vi "2DRandomInterp.vi"() -> ()   [LabVIEW 2016]
uses:
  <vilib>/gmath/interp.llb/Interpolate 2D (2d X,Y).vi
  <vilib>/picture/3D Picture Control/Object/Create Object (drawable).vi
  <vilib>/picture/3D Picture Control/Helpers/Apply Texture (no reference).vi
  <vilib>/gmath/NI_Gmath.lvlib
  <vilib>/picture/3D Picture Control/NI_3D Picture Control.lvlib
  <vilib>/picture/3D Picture Control/Object/Add Object (no reference).vi
panel:
  out "3D Picture":refnum<vi>(3d-picture)
  in  "x":i32
  in  "y":i32
  in  "ntimes":i32=5
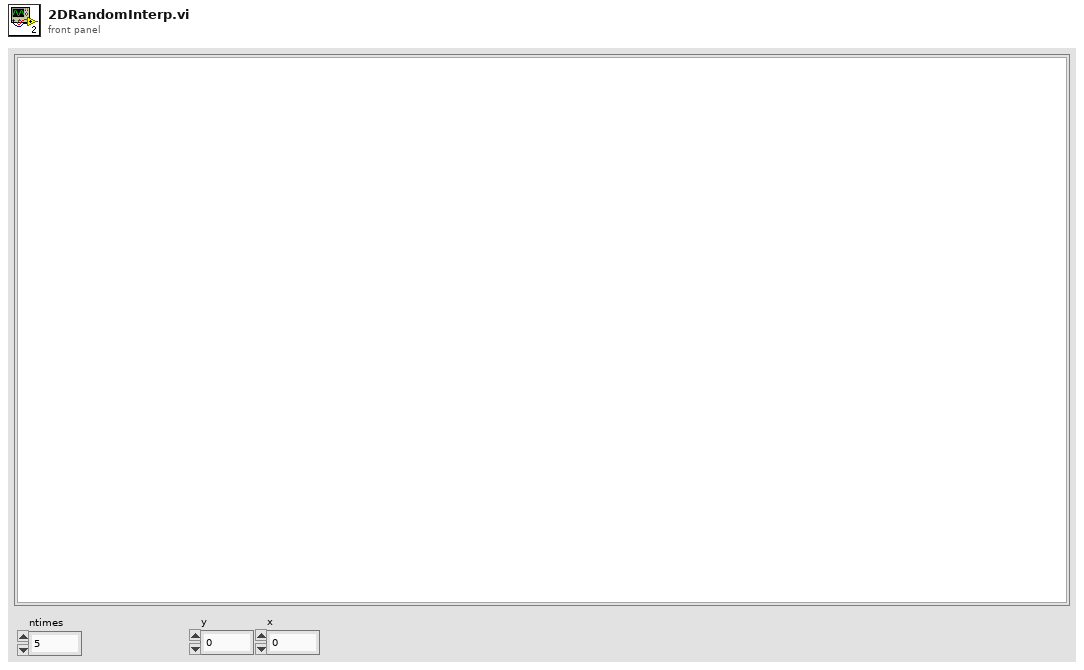
[diagram p1: front panel]
types:
  T1 = enum16{"As a Decal", "With Modulation", "With Blending", "As a replacement"}
  T2 = typedef "imagedata.ctl" = cluster{"image type":i32, "image depth":i32, "image":u8[], "mask":u8[], "colors":u32[], "Rectangle":cluster{"left":i16, "top":i16, "right":i16, "bottom":i16}}
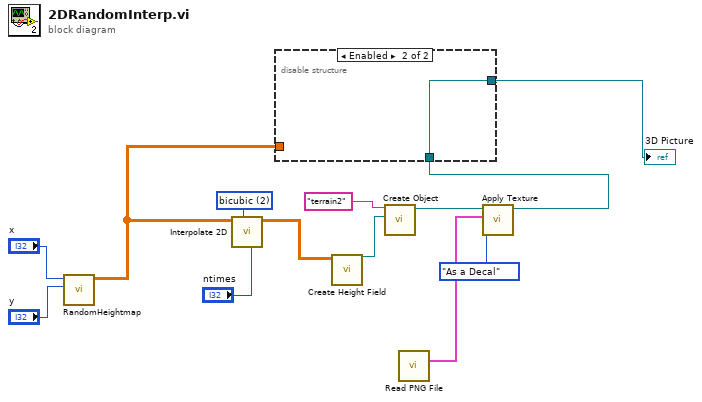
[diagram p0: block diagram]
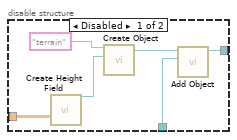
[diagram p2: hidden frame]
diagram:
  w13 = 2 items=["nearest", "bilinear", "bicubic", "bicubic spline"] ("method")
  n1 = call "RandomHeightmap.vi"("y"="y", "x"="x") -> ("Array"=w9:dbl[][])  [unwired: 9 in]
  n2 = call-poly <vilib>:"Interpolate 2D.vi"("ntimes"="ntimes", "method"=w13, "Z"=w9) -> ("zi"=w6:dbl[][])  [unwired: 5 in, 3 out]
  n3 = call <vilib>:"Create Height Field.vi"("Data"=w6) -> ("New Height Field Refnum"=w7:refnum<vi>)  [unwired: 9 in, 1 out]
  n4 = call-poly <vilib>:"Create Object.vi"("Geometry"=w7, "Name"="terrain2") -> ("Scene:New Object"=w4:refnum<vi>)  [unwired: 8 in, 1 out]
  n5 = call <vilib>:"Read PNG File.vi"() -> ("image data"=w2:T2)  [unwired: 9 in, 2 out]
  n6 = call-poly <vilib>:"Apply Texture.vi"("Apply Mode"=T1."As a Decal", "Image Data"=w2, "Scene Object In"=w4) -> ("Scene Object Out"=w3:refnum<vi>)  [unwired: 7 in, 1 out]
  n7 = disable-structure shown="Enabled" {
    disable-tunnel: w9 -> [w19 _]
    disable-tunnel: w3 -> [w15 w20]
    disable-tunnel: [w14 w20] -> w5
    frame Disabled {
      n8 = call <vilib>:"Create Height Field.vi"("Data"=w19) -> ("New Height Field Refnum"=w18:refnum<vi>)  [unwired: 9 in, 1 out]
      n9 = call-poly <vilib>:"Create Object.vi"("Geometry"=w18, "Name"="terrain") -> ("Scene:New Object"=w16:refnum<vi>)  [unwired: 8 in, 1 out]
      n10 = call-poly <vilib>:"Add Object.vi"("New Object In"=w15, "Scene Object In"=w16) -> ("Scene Object Out"=w14:refnum<vi>)  [unwired: 8 in, 1 out]
    }
    frame Enabled {
    }
  }
  "3D Picture" <- w5
